vi "Stacked Shift Registers.vi"() -> ()   [LabVIEW 2023]
panel:
  out "Sequentially Greater":bool
  out "Previous Number":dbl
  out "Numeric":i32
  in  "stop":bool
  out "number (0 to 1)":dbl
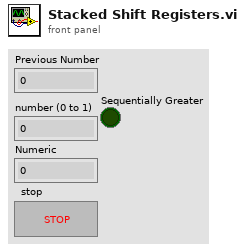
[diagram p1: front panel]
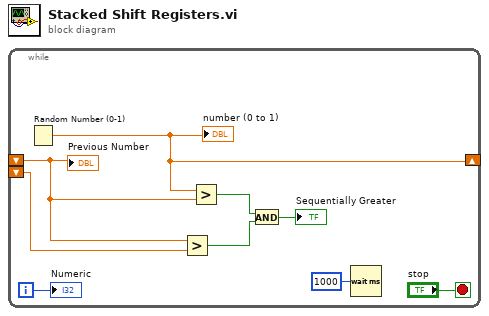
[diagram p0: block diagram]
diagram:
  n1 = while {
    shift-right: [w5] -> _
    shift-left: _ -> [w4]
    shift-left: _ -> [w6]
    i -> [w8]
    stop <- "stop" stop-if-true
    n2 = Random Number (0-1)() -> (number: 0 to 1=w5:dbl)
    "number (0 to 1)" <- w5
    n3 = Greater?(x=w4, y=w6) -> (0:w2:bool)
    n4 = Greater?(x=w5, y=w4) -> (0:w3:bool)
    n5 = And(x=w3, y=w2) -> (x .and. y?=→"Sequentially Greater":bool)
    n6 = Wait (ms)(milliseconds to wait=u32 1000) -> ()  [unwired: 1 out]
    "Numeric" <- w8
    "Previous Number" <- w4
  }
